vi "benchmarks_fileMD5.vi"() -> ()   [LabVIEW 2013]
uses:
  MD5/MD5.lvclass
  <vilib>/Analysis/baseanly.llb/Mean (DBL).vi
  MD5/Enqueue File.vi
  MD5/pad.vi
  MD5/MD5.lvlib
  <vilib>/Analysis/NI_AALBase.lvlib
panel:
  out "equal hashes":bool
  out "% gain":dbl
  out "LVOS":dbl
  out "NI":dbl
  in  "filepath":path
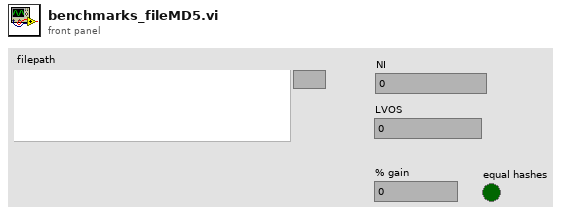
[diagram p1: front panel]
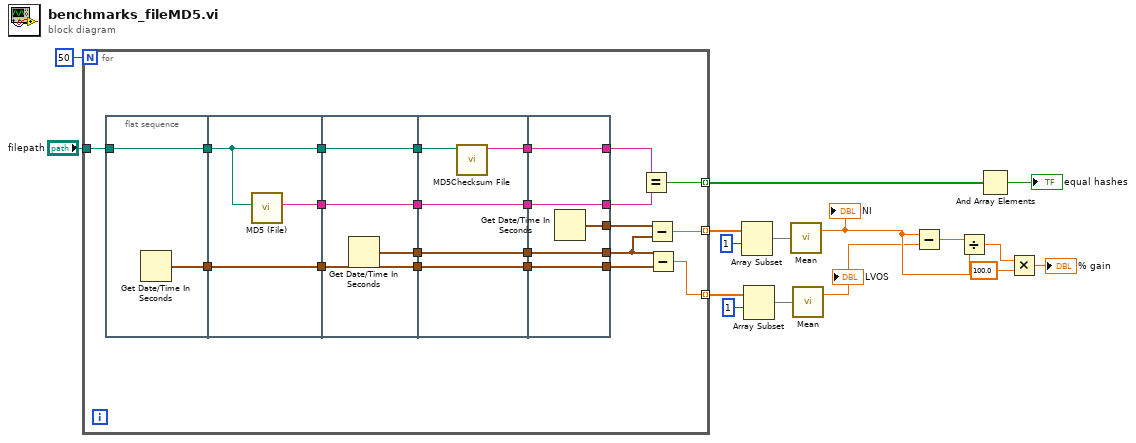
[diagram p0: block diagram]
diagram:
  n1 = for {
    N: 50 -> [_]
    tunnel: "filepath" -> [w25]
    tunnel: [w19] -> w15 mode=indexing
    tunnel: [w18] -> w8 mode=indexing
    tunnel: [w17] -> w7 mode=indexing
    n2 = flat-sequence {
      tunnel: w25 -> [w40]
      tunnel: [w40] -> w38
      tunnel: [w39] -> w37
      tunnel: [w43] -> w36
      tunnel: w38 -> [w43]
      tunnel: w37 -> [w42]
      tunnel: [w42] -> w35
      tunnel: [w41] -> w34
      tunnel: w36 -> [w47]
      tunnel: [w47] -> w33
      tunnel: [w46] -> w32
      tunnel: [w45] -> w31
      tunnel: w35 -> [w45]
      tunnel: [w44] -> w30
      tunnel: w34 -> [w44]
      tunnel: w33 -> [w52]
      tunnel: [w51] -> w29
      tunnel: w32 -> [w51]
      tunnel: [w50] -> w28
      tunnel: w31 -> [w50]
      tunnel: [w49] -> w27
      tunnel: [w48] -> w26
      tunnel: w30 -> [w48]
      tunnel: [w57] -> w23
      tunnel: w29 -> [w57]
      tunnel: [w56] -> w22
      tunnel: w28 -> [w56]
      tunnel: [w55] -> w24
      tunnel: [w54] -> w21
      tunnel: w27 -> [w54]
      tunnel: [w53] -> w20
      tunnel: w26 -> [w53]
      frame #0 {
        n3 = Get Date/Time In Seconds() -> (seconds since 1Jan1904=w39:timestamp)
      }
      frame #1 {
        n4 = call "MD5 (File).vi"("filepath"=w43) -> ("MD5 hash"=w41:string)  [unwired: 10 in]
      }
      frame #2 {
        n5 = Get Date/Time In Seconds() -> (seconds since 1Jan1904=w46:timestamp)
      }
      frame #3 {
        n6 = call <vilib>:"MD5Checksum File.vi"("Path"=w52) -> ("MD5 message-digest"=w49:string)  [unwired: 9 in, 1 out]
      }
      frame #4 {
        n7 = Get Date/Time In Seconds() -> (seconds since 1Jan1904=w55:timestamp)
      }
    }
    n8 = Equal?(x=w21, y=w20) -> (x = y?=w19:bool)
    n9 = Subtract(x=w24, y=w23) -> (x-y=w18:dbl)
    n10 = Subtract(x=w23, y=w22) -> (x-y=w17:dbl)
  }
  n11 = Array Subset(array=w8, index=1) -> (w11:dbl[])  [unwired: 1 in]
  n12 = Array Subset(array=w7, index=1) -> (w10:dbl[])  [unwired: 1 in]
  n13 = call-poly <vilib>:"Mean.vi"("X"=w11) -> ("mean"=w3:dbl)  [unwired: 1 out]
  "NI" <- w3
  n14 = call-poly <vilib>:"Mean.vi"("X"=w10) -> ("mean"=w2:dbl)  [unwired: 1 out]
  "LVOS" <- w2
  n15 = Subtract(x=w3, y=w2) -> (x-y=w6:dbl)
  n16 = Divide(x=w6, y=w3) -> (x/y=w4:dbl)
  n17 = And Array Elements(Boolean array=w15) -> (logical AND=→"equal hashes":bool)
  n18 = Multiply(x=w4, y=100.0) -> (x*y=→"% gain":dbl)
